vi "Compare Calls.vi"(8 "error in (no error)":errorcluster, 9 "VI Call 2":refnum<class "VI Call.lvclass">, 10 "VI Call 1":refnum<class "VI Call.lvclass">, 11 "Identical Inputs Comparator In":refnum<class "Identical Inputs Comparator.lvclass">) -> (0 "error out":errorcluster, 1 "Description":string, 2 "Equal?":bool)   [LabVIEW 2020, in "Identical Inputs Comparator.lvclass"]
uses:
  Identical Inputs Comparator.lvclass
  Call/VI Call.lvclass
  Mock/Mock.lvclass
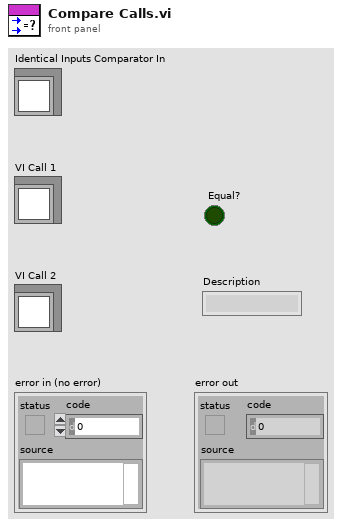
[diagram p1: front panel]
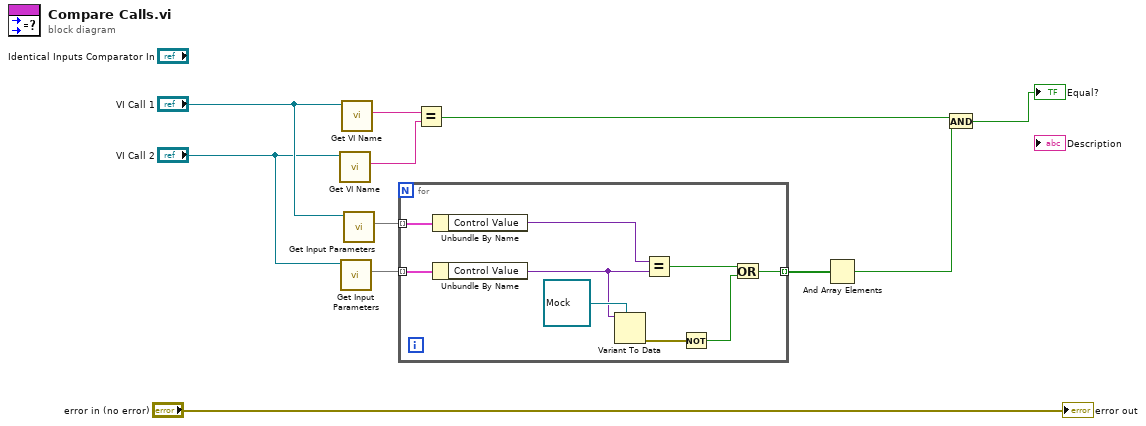
[diagram p0: block diagram]
diagram:
  n1 = call-dynamic "Get VI Name.vi"("VI Call in"="VI Call 2") -> ("VI Name"=w8:string)  [unwired: 9 in, 1 out]
  n2 = call-dynamic "Get Input Parameters.vi"("VI Call In"="VI Call 2") -> ("Input Parameters"=w5:map{string, variant})  [unwired: 9 in, 1 out]
  n3 = call-dynamic "Get VI Name.vi"("VI Call in"="VI Call 1") -> ("VI Name"=w9:string)  [unwired: 9 in, 1 out]
  n4 = call-dynamic "Get Input Parameters.vi"("VI Call In"="VI Call 1") -> ("Input Parameters"=w6:map{string, variant})  [unwired: 9 in, 1 out]
  n5 = for {
    tunnel: w6 -> [w20] mode=indexing
    tunnel: w5 -> [w19] mode=indexing
    tunnel: [w14] -> w4 mode=indexing
    n6 = Unbundle By Name(w20) -> ("Control Value"=w17:variant)
    n7 = Unbundle By Name(w19) -> ("Control Value"=w15:variant)
    n8 = Variant To Data(type=refnum<class "Mock.lvclass"> refnum ("Mock.lvclass"), Variant=w15) -> (error out=w13:errorcluster)  [unwired: 1 in, 1 out]
    n9 = Equal?(x=w17, y=w15) -> (x = y?=w18:bool)
    n10 = Not(x=w13) -> (.not. x?=w12:bool)
    n11 = Or(x=w18, y=w12) -> (x .or. y?=w14:bool)
  }
  n12 = Equal?(x=w9, y=w8) -> (x = y?=w1:bool)
  n13 = And Array Elements(Boolean array=w4) -> (logical AND=w3:bool)
  n14 = And(x=w1, y=w3) -> (x .and. y?=→"Equal?":bool)
  "error out" <- "error in (no error)"
